vi "Insert Case Structure.vi"(0 "Test Executive Ref":refnum<data-value>, 1 "Name":string, 2 "Unique ID":string, 3 "Insertion Index":i32=-1, 4 "Assertions":refnum<class "Assert.lvclass">[](array[class]), 5 "error in (no error)":errorcluster, 6 "Parent ID":string, 7 "X Variables":string[](array[string]), 9 "Y Variables":string[](array[string]), 11 "Conditional Branches":string[](array[string]), 13 "\"Else\" Conditional Branch":string) -> (12 "Unique ID out":string, 14 "Test Executive Ref out":refnum<data-value>, 17 "Replaced?":bool, 19 "error out":errorcluster)   [LabVIEW 2019, in "Test Executive.lvlib" / "TestExecutive Ref.lvclass"]
uses:
  <vilib>/gpm_packages/@cs/test-executive/Source/Test Executive/TestExecutive Ref/TestExecutive Ref.lvclass
  <vilib>/gpm_packages/@cs/test-executive/Source/Test Executive/ITestExecutive/ITest Executive.lvclass
  <vilib>/gpm_packages/@cs/run-time-assertions/Source/Assert/Assert.lvclass
  <vilib>/Utility/error.llb/Error Cluster From Error Code.vi
  <vilib>/ErrorRing/Error Ring.xnode
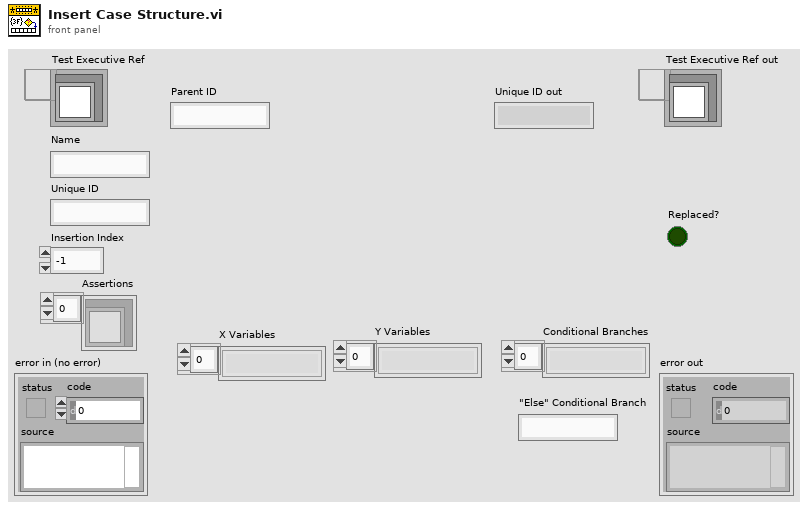
[diagram p1: front panel]
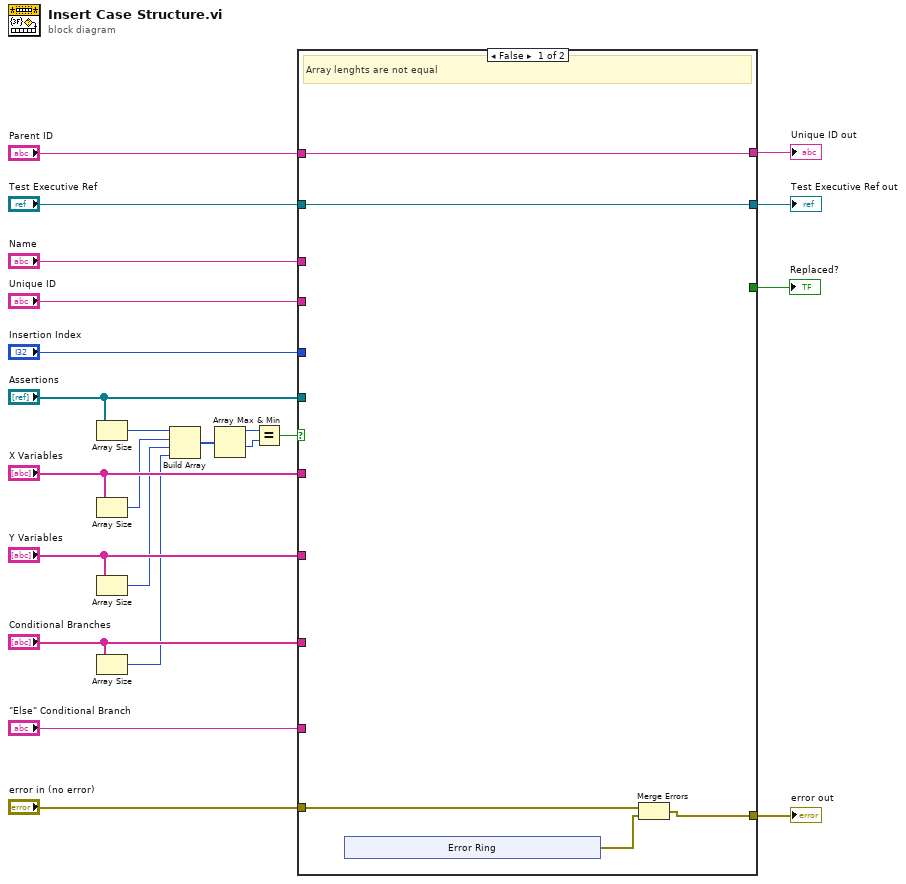
[diagram p0: block diagram]
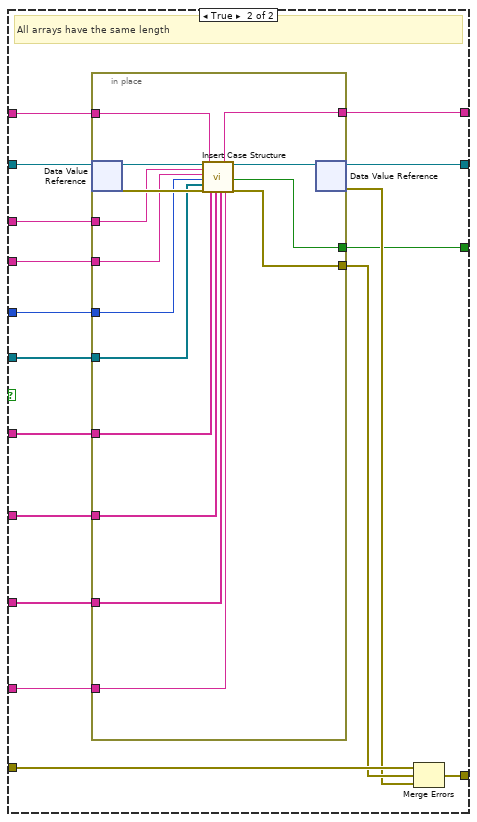
[diagram p2: hidden frame]
diagram:
  n1 = Array Size(array="Assertions") -> (size(s)=w8:i32)
  n2 = Array Size(array="X Variables") -> (size(s)=w7:i32)
  n3 = Array Size(array="Y Variables") -> (size(s)=w6:i32)
  n4 = Array Size(array="Conditional Branches") -> (size(s)=w5:i32)
  n5 = Build Array(w8, w7, w6, w5) -> (w4:i32[])
  n6 = Array Max & Min(array=w4) -> (max value=w3:i32, min value=w2:i32)  [unwired: 2 out]
  n7 = Equal?(x=w3, y=w2) -> (x = y?=w1:bool)
  n8 = case shown="False" w1 {
    tunnel: "Test Executive Ref" -> [w27 w50]
    tunnel: "Parent ID" -> [w28 w49]
    tunnel: "Name" -> [_ w48]
    tunnel: "Insertion Index" -> [_ w47]
    tunnel: [w27 w46] -> w19
    tunnel: [w28 w45] -> w18
    tunnel: "error in (no error)" -> [w26 w44]
    tunnel: [w24 w41] -> w16
    tunnel: "Unique ID" -> [_ w40]
    tunnel: [_ w39] -> w14
    tunnel: "\"Else\" Conditional Branch" -> [_ w38]
    tunnel: "Assertions" -> [_ w37]
    tunnel: "X Variables" -> [_ w36]
    tunnel: "Y Variables" -> [_ w35]
    tunnel: "Conditional Branches" -> [_ w34]
    frame False {
      # "Array lenghts are not equal"
      n9 = xnode "Error Ring"() -> ("error out"=w25:errorcluster)
      n10 = Merge Errors(w26, w25) -> (w24:errorcluster)
    }
    frame True {
      # "All arrays have the same length"
      n11 = in-place {
        in-place-border: w49 -> [w58]
        in-place-border: w48 -> [w61]
        in-place-border: w40 -> [w60]
        in-place-border: w47 -> [w59]
        in-place-border: [w57] -> w45
        in-place-border: [w62] -> w43
        in-place-border: [w56] -> w39
        in-place-border: w37 -> [w55]
        in-place-border: w36 -> [w54]
        in-place-border: w35 -> [w53]
        in-place-border: w34 -> [w52]
        in-place-border: w38 -> [w51]
        n12 = in-place-dvr #1(w50) -> (w65:refnum<class "ITest Executive.lvclass">, w63:errorcluster)
        n13 = call-dynamic "Insert Case Structure.vi"("ITest Executive in"=w65, "Name"=w61, "Unique ID"=w60, "Insertion Index"=w59, "Assertions"=w55, "error in (no error)"=w63, "Parent ID"=w58, "X Variables"=w54, "Y Variables"=w53, "Conditional Branches"=w52, "\"Else\" Conditional Branch"=w51) -> ("Unique ID out"=w57:string, "ITest Executive out"=w64:refnum<class "ITest Executive.lvclass">, "Replaced?"=w56:bool, "error out"=w62:errorcluster)  [unwired: 5 in]
        n14 = in-place-dvr #1(w64) -> (w46:refnum<data-value>, w42:errorcluster)
      }
      n15 = Merge Errors(w44, w43, w42) -> (w41:errorcluster)
    }
  }
  "Test Executive Ref out" <- w19
  "error out" <- w16
  "Unique ID out" <- w18
  "Replaced?" <- w14
